vi "HJ -Set group jerk.vi"(0 "Address / Port":i16=1 min=1 max=31 step=1, 1 "Group #":i8=1 min=1 max=6 step=1, 2 "Vectorial jerk\nset":dbl format="%.2f", 3 "error in":errorcluster, 4 "Action":bool) -> (5 "Vectorial jerk\nread":string, 6 "error out":errorcluster)   [LabVIEW 2014]
panel:
  # "Read"
  # "Write"
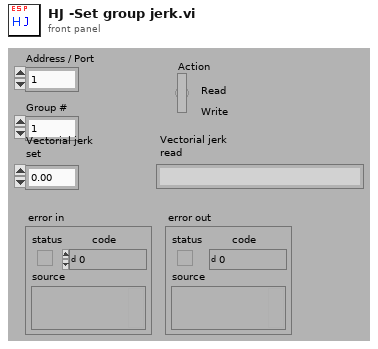
[diagram p1: front panel]
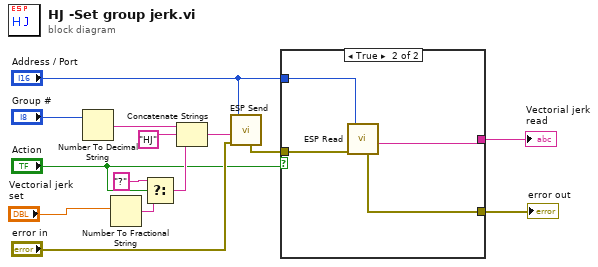
[diagram p0: block diagram]
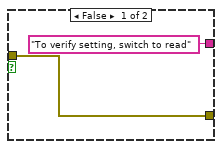
[diagram p2: hidden frame]
diagram:
  n1 = Number To Decimal String(number="Group #") -> (decimal integer string=w13:string)  [unwired: 1 in]
  n2 = Number To Fractional String(number="Vectorial jerk\nset") -> (F-format string=w9:string)  [unwired: 3 in]
  n3 = Select(t="?", s="Action", f=w9) -> (s? t:f=w10:string)
  n4 = Concatenate Strings(w13, "HJ" ("Substring"), w10) -> (w11:string)
  n5 = call "ESP Send.vi"("Address / Port"="Address / Port", "Command String"=w11, "error in"="error in") -> ("error out"=w4:errorcluster)  [unwired: 5 in]
  n6 = case shown="True" "Action" {
    tunnel: "Address / Port" -> [_ w20]
    tunnel: w4 -> [w16 w19]
    tunnel: [w16 w18] -> w3
    tunnel: ["To verify setting, switch to read" w17] -> w1
    frame False {
    }
    frame True {
      n7 = call "ESP Read.vi"("Address / Port"=w20, "error in"=w19) -> ("error out"=w18:errorcluster, "Response String"=w17:string)  [unwired: 5 in]
    }
  }
  "error out" <- w3
  "Vectorial jerk\nread" <- w1
